vi "load data.vi"(7 "Append dataset":bool, 9 "show files":T1(array[cluster])=[{"String"="20120217.012", "Boolean"=TRUE, "begin"=15, "length"=10000, "y weight"=1.0}], 10 "existing file numbers":string[](array[string]), 11 "existing data cluster":cluster{"array type (2D Dbl)":dbl[][]}[](array[cluster])) -> (1 "show files out":T1(array[cluster])=[{"String"="20120217.012", "Boolean"=TRUE, "begin"=15, "length"=10000, "y weight"=1.0}], 2 "data names":string[](array[string]), 3 "data cluster":cluster{"all data":dbl[][]}[](array[cluster]))   [LabVIEW 2025]
uses:
  <vilib>/Utility/file.llb/Read Delimited Spreadsheet (DBL).vi
panel:
  in  "data view":bool
  in  "Done":bool
  out "# of datasets":i32
  in  "numbered file":T2={"FILE HEADER"="20120217", "FROM"="012", "TO"="012", "Excluding\nFrom"="", "Excluding\nTo"="", "Start Loading\ndata files"=FALSE, "cancel"=FALSE}
  in  "Cancel button":bool
  in  "Import Menu":T3(ring)
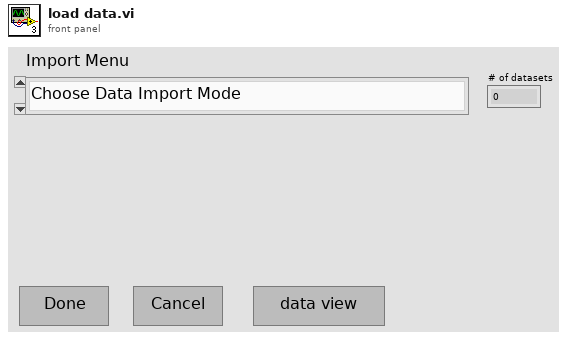
[diagram p1: front panel]
types:
  T1 = cluster{"String":string, "Boolean":bool, "begin":u32, "length":u32, "y weight":dbl}[]
  T2 = cluster{"FILE HEADER":string, "FROM":string, "TO":string, "Excluding\nFrom":string, "Excluding\nTo":string, "Start Loading\ndata files":bool, "cancel":bool}
  T3 = enum16{"Choose Data Import Mode", "Numbered NML Data Acq files saved in the drive", "Import current data being taken", "Manual selection of text file(s) ", "Manual Input of single XY plot(s)", "Manual Input of a worksheet", "Select files from a folder", "Delete Datasets"}
  T4 = enum16{"Choose Data Import Mode", "Numbered NML Data Acq files saved in the drive", "Import current data being taken", "Manual selection of text file(s) ", "Manual Input of single XY plot(s)", "Manual Input of a worksheet"}
  T5 = enum16{"Choose Data Import Mode", "Numbered NML Data Acq files saved in the drive", "Import current NML Data Acq being taken", "Manual selection of text file(s) ", "Manual Input of XY arrays", "Manual Input of a worksheet"}
  T6 = cluster{"String":string, "data view":bool, i32, i32, "new entry identier":dbl}
  T7 = cluster{"file name":string, "data view":bool, i32, i32, "new entry identier":dbl}
  T8 = cluster{"file name":string, "data view":bool, i32, i32, "new entry identier":dbl}[]
  T9 = cluster{"name":string, "data view":bool, i32, i32, "new entry identier":dbl}
  T10 = cluster{"dataset name (option)":string, "data view":bool, i32, i32, "new entry identier":dbl}
  T11 = cluster{"data set names":string, "data view":bool, i32, i32, "new entry identier":dbl}
  T12 = enum16{"Left Button", "Center Button", "Right Button", "Window Close"}
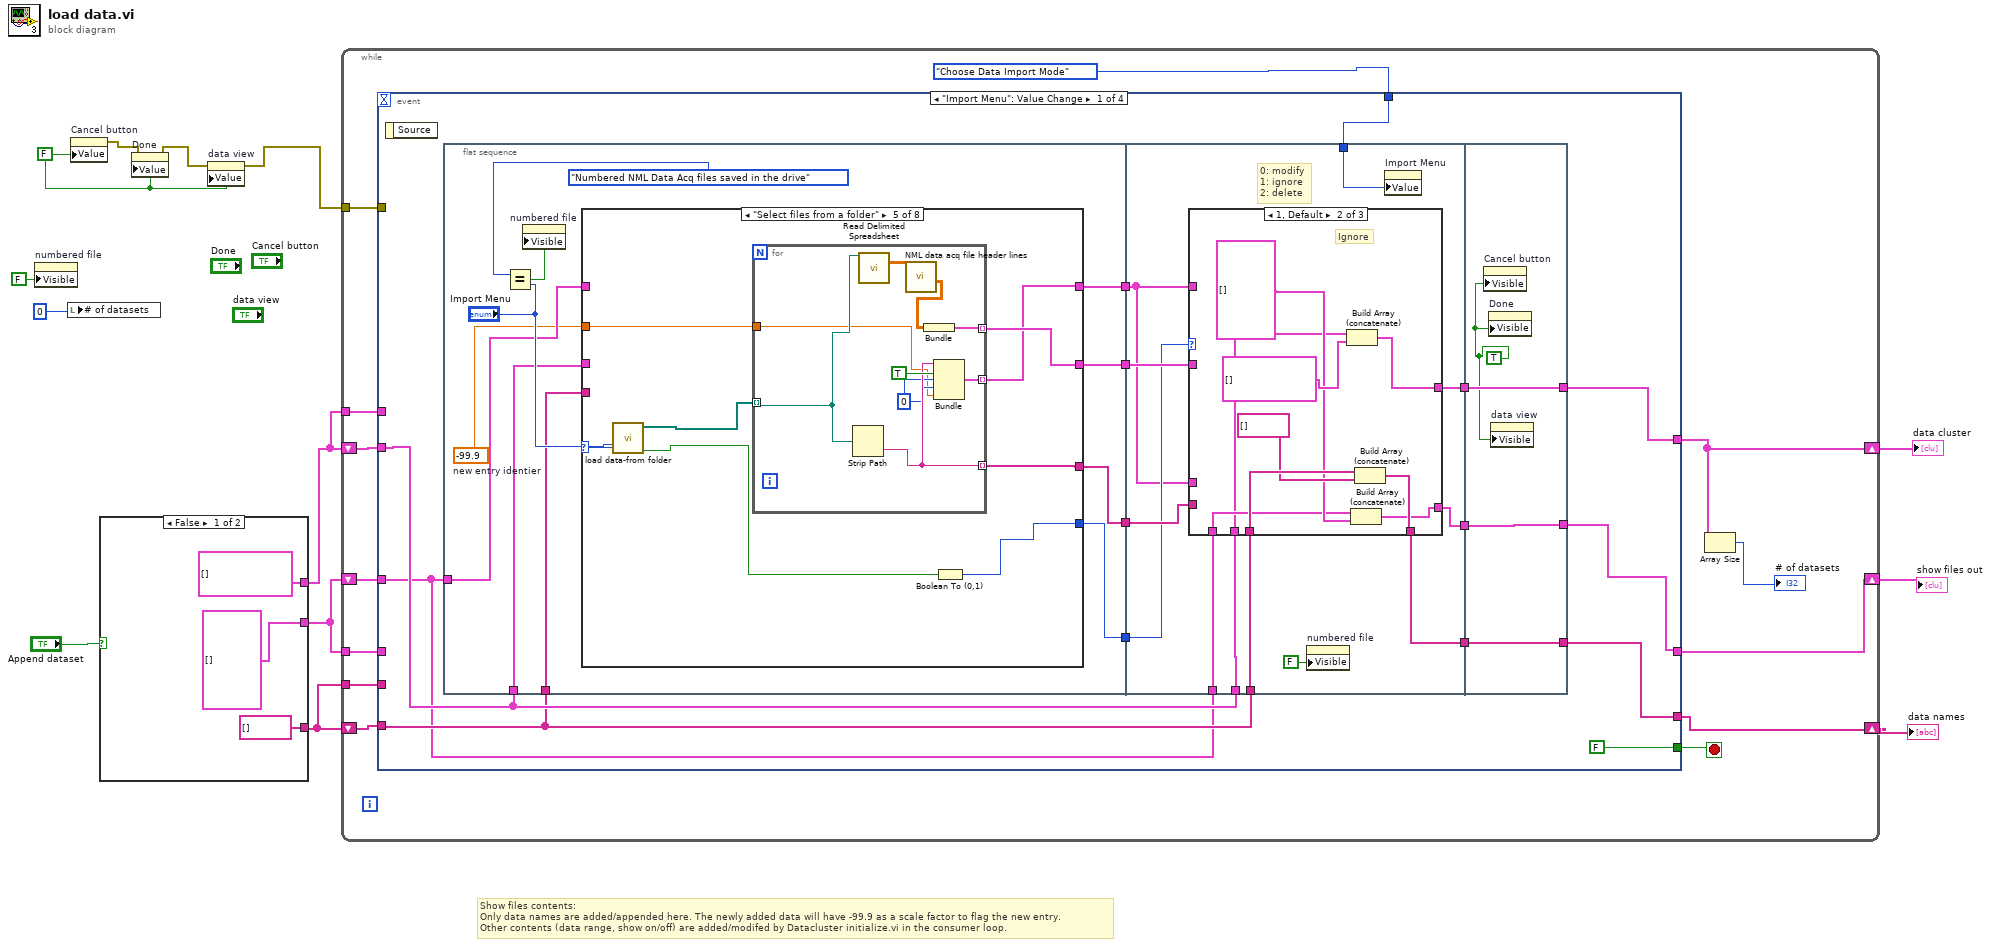
[diagram p0: block diagram]
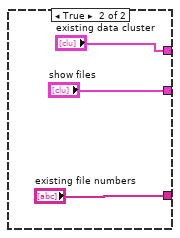
[diagram p2: hidden frame]
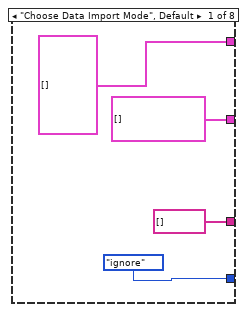
[diagram p3: hidden frame]
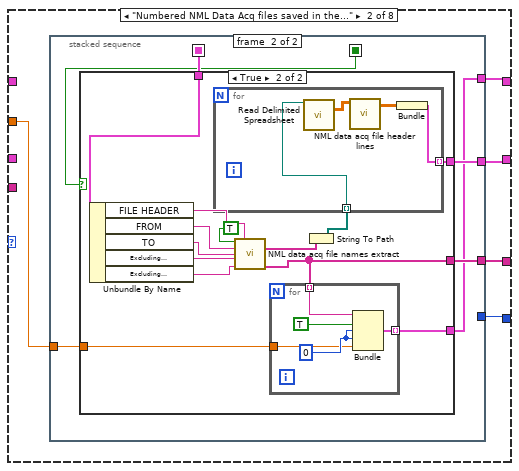
[diagram p4: hidden frame]
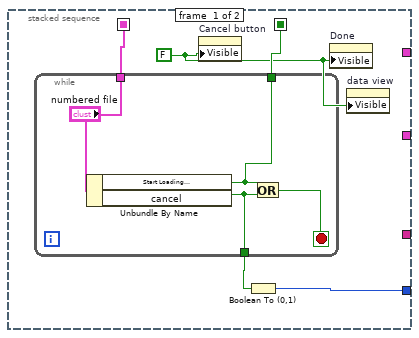
[diagram p5: hidden frame]
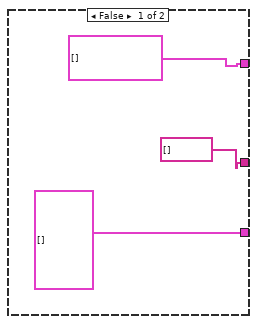
[diagram p6: hidden frame]
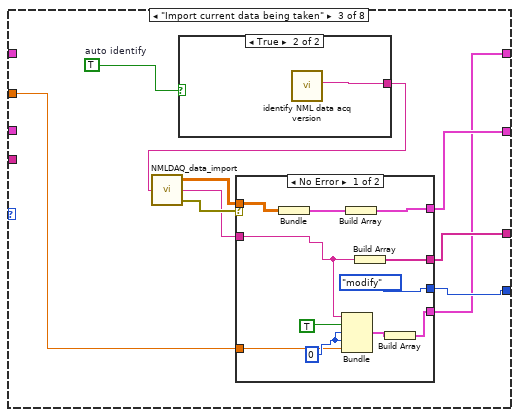
[diagram p7: hidden frame]
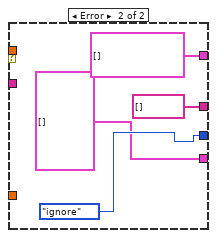
[diagram p8: hidden frame]
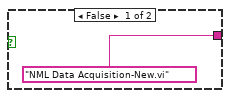
[diagram p9: hidden frame]
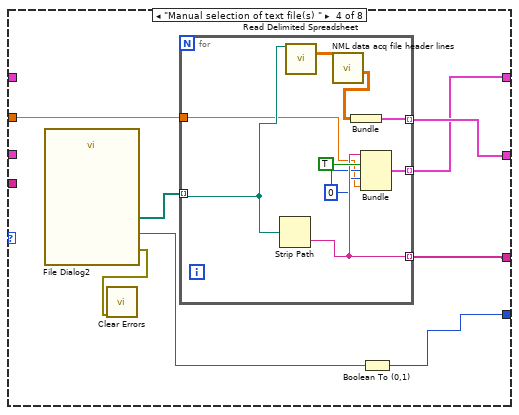
[diagram p10: hidden frame]
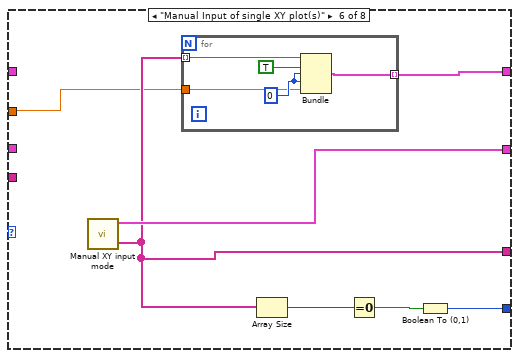
[diagram p11: hidden frame]
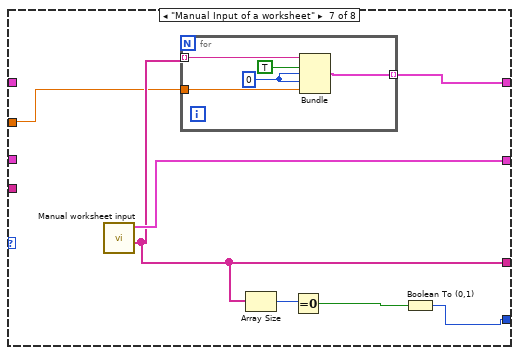
[diagram p12: hidden frame]
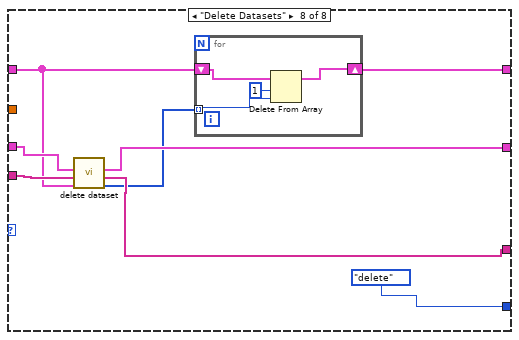
[diagram p13: hidden frame]
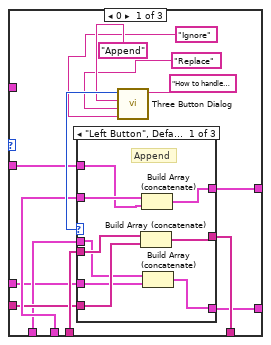
[diagram p14: hidden frame]
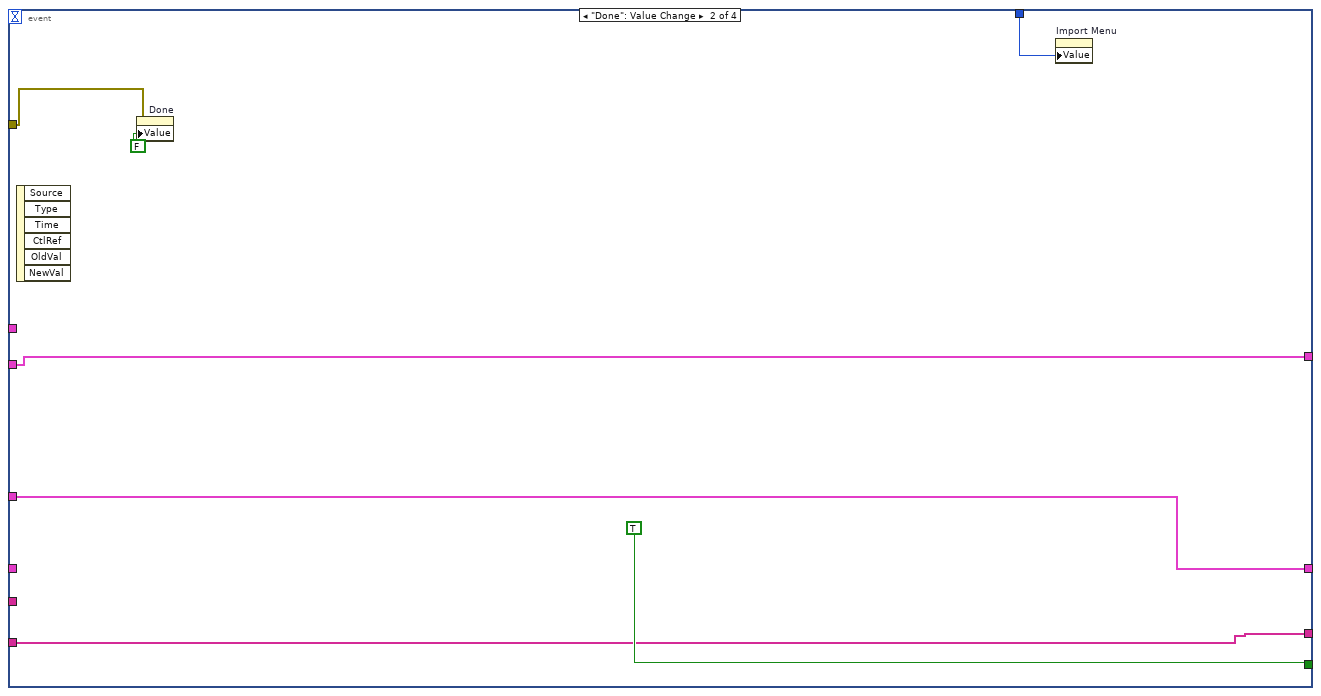
[diagram p18: hidden frame]
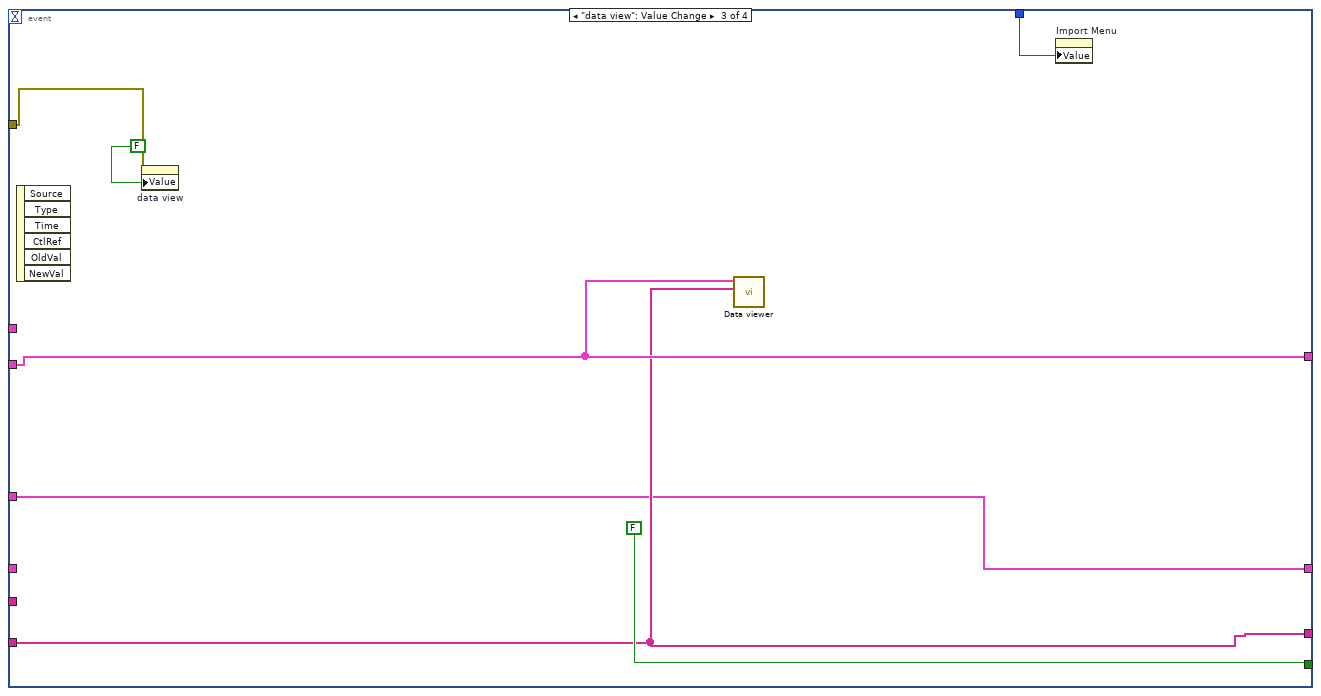
[diagram p19: hidden frame]
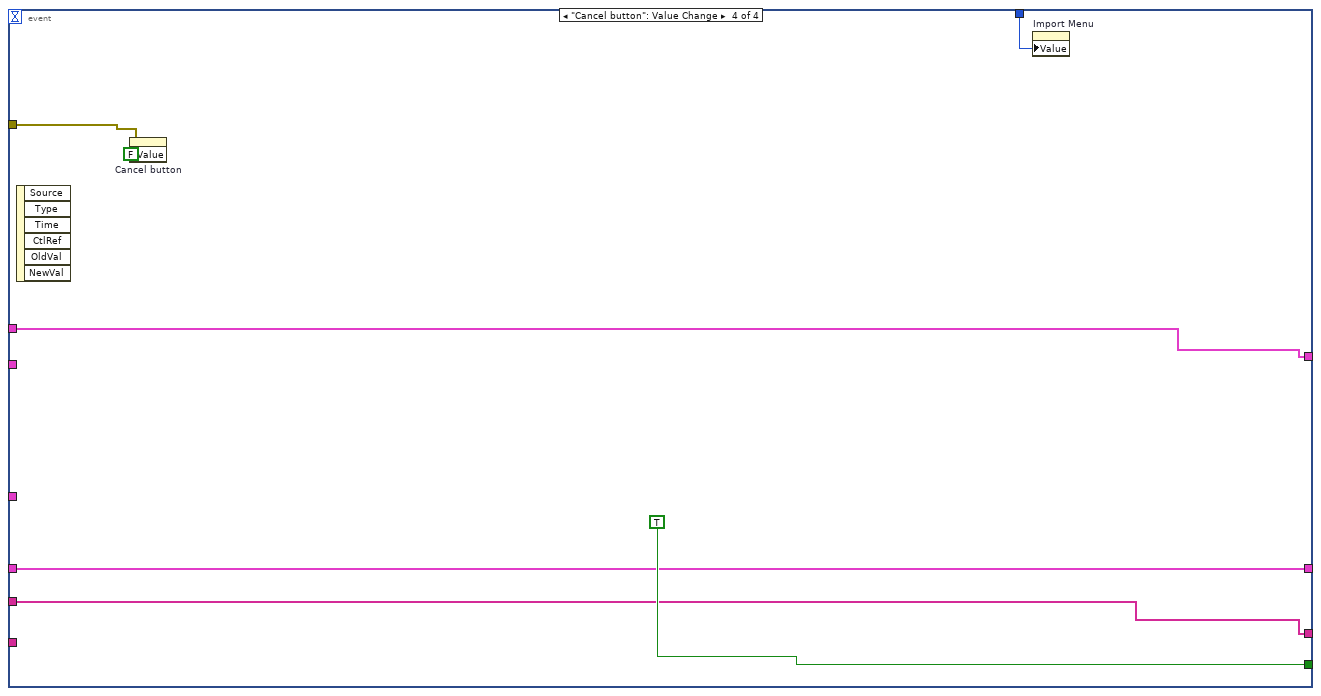
[diagram p20: hidden frame]
diagram:
  w5 = FALSE ("Value (Signaling)")
  # "Show files contents:\nOnly data names are added/appended here. The newly added data will have -99.9 as a scale factor to flag the new entry.\nOther contents (data range, show on/off) are added/modifed by Datacluster initialize.vi in the consumer loop."
  n1 = property on="numbered file" class="Clust"("Visible"=FALSE) -> ()  [unwired: 2 in, 2 out]
  n2 = local write "# of datasets"(0 ("# of data files")) -> ()
  n3 = property on="Cancel button" class="Bool (strict)"("Value"=w5) -> (error out=w8:errorcluster)  [unwired: 2 in, 1 out]
  n4 = case shown="False" "Append dataset" {
    tunnel: [cluster{"array type (2D Dbl)":dbl[][]}[] [] ("existing data cluster") "existing data cluster"] -> w4
    tunnel: [string[] [] ("existing file numbers") "existing file numbers"] -> w3
    tunnel: [T1 [] ("show files") "show files"] -> w2
    frame False {
    }
    frame True {
    }
  }
  n5 = property on="Done" class="Bool (strict)"(error in=w8, "Value"=w5) -> (error out=w7:errorcluster)  [unwired: 1 in, 1 out]
  n6 = property on="data view" class="Bool (strict)"(error in=w7, "Value"=w5) -> (error out=w6:errorcluster)  [unwired: 1 in, 1 out]
  n7 = while {
    shift-right: [w27] -> w10
    shift-left: w4 -> [w31]
    shift-right: [w28] -> w11
    shift-left: w3 -> [w29]
    tunnel: w6 -> [w26]
    tunnel: w4 -> [w24]
    tunnel: w3 -> [w23]
    shift-right: [w20] -> w1
    shift-left: w2 -> [w22]
    tunnel: w2 -> [w21]
    stop <- w32 stop-if-true
    n8 = event shown="[0] \"Import Menu\": Value Change" {
      selector: _ -> [_ _ _ _]
      dyn-events: _ -> [_ _ _ _]
      timeout: _ -> [_ _ _ _]
      tunnel: [FALSE TRUE FALSE TRUE] -> w32
      tunnel: [w46 w266 w272 w277] -> w27
      tunnel: w31 -> [w38 w266 w272 _]
      tunnel: [w45 w265 w271 w276] -> w28
      tunnel: w29 -> [w37 w265 w271 _]
      tunnel: w26 -> [_ w264 w269 w280]
      tunnel: T4."Choose Data Import Mode" ("Import Menu") -> [w44 w262 w273 w278]
      tunnel: w24 -> [_ _ _ w277]
      tunnel: w23 -> [_ _ _ w276]
      tunnel: w22 -> [w33 w261 w268 _]
      tunnel: w21 -> [_ _ _ w275]
      tunnel: [w35 w261 w268 w275] -> w20
      event "Import Menu": Value Change {
        n9 = event-data() -> ()  [unwired: 1 in, 1 out]
        n10 = flat-sequence {
          tunnel: [w56] -> w43
          tunnel: [w55] -> w42
          tunnel: [w51] -> w39
          tunnel: w38 -> [w53]
          tunnel: w37 -> [w52]
          tunnel: [w50] -> w36
          tunnel: w33 -> [w49]
          tunnel: w43 -> [w212]
          tunnel: w42 -> [w213]
          tunnel: w38 -> [w215]
          tunnel: w37 -> [w214]
          tunnel: w44 -> [w208]
          tunnel: [w211] -> w41
          tunnel: [w210] -> w40
          tunnel: w39 -> [w207]
          tunnel: w36 -> [w204]
          tunnel: [w206] -> w34
          tunnel: w33 -> [w205]
          tunnel: [w259] -> w45
          tunnel: [w260] -> w46
          tunnel: w41 -> [w260]
          tunnel: w40 -> [w259]
          tunnel: [w257] -> w35
          tunnel: w34 -> [w257]
          frame #0 {
            w48 = -99.9  # new entry identier
            n11 = Equal?(x=T5."Numbered NML Data Acq files saved in the drive", y="Import Menu") -> (x = y?=w54:bool)
            n12 = property on="numbered file" class="Clust"("Visible"=w54) -> ()  [unwired: 2 in, 2 out]
            n13 = case shown="\"Select files from a folder\"" "Import Menu" {
              tunnel: [cluster{"array type (2D Dbl)":dbl[][]}[] [] ("Data clusters") w67 w111 w142 w158 w174 w186 w196] -> w56
              tunnel: [string[] [] ("file numbers") w66 w112 w140 w157 w170 w181 w195] -> w55
              tunnel: [enum16{"modify", "ignore", "delete"}."ignore" ("Enum") w65 w110 w137 w156 w171 w183 enum16{"modify", "ignore", "delete"}."delete" ("Enum")] -> w51
              tunnel: w53 -> [_ _ _ _ _ _ _ w197]
              tunnel: w52 -> [_ _ _ _ _ _ _ w198]
              tunnel: w49 -> [_ _ _ _ _ _ _ w193]
              tunnel: [T1 [] ("show files") w64 w109 w136 w155 w169 w182 w192] -> w50
              tunnel: w48 -> [_ w63 w108 w135 w154 w168 w180 _]
              frame "Choose Data Import Mode", Default {
              }
              frame "Numbered NML Data Acq files saved in the drive" {
                n14 = stacked-sequence {
                  seq-local: [w72 _] -> [_ w81]
                  seq-local: [w71 _] -> [_ w79]
                  tunnel: [_ w82] -> w67
                  tunnel: [_ w80] -> w66
                  tunnel: [w69 _] -> w65
                  tunnel: [_ w78] -> w64
                  tunnel: w63 -> [_ w77]
                  frame #0 {
                    w68 = FALSE ("Visible")
                    n15 = while {
                      tunnel: ["numbered file"] -> w72
                      tunnel: [w74] -> w71
                      tunnel: [w73] -> w70
                      stop <- w75 stop-if-true
                      n16 = Unbundle By Name("numbered file") -> ("Start Loading\ndata files"=w74:bool, "cancel"=w73:bool)
                      n17 = Or(x=w74, y=w73) -> (x .or. y?=w75:bool)
                    }
                    n18 = property on="Cancel button" class="Bool (strict)"("Visible"=w68) -> ()  [unwired: 2 in, 2 out]
                    n19 = Boolean To (0,1)(Boolean=w70) -> (0, 1=w69:i16)
                    n20 = property on="Done" class="Bool (strict)"("Visible"=w68) -> ()  [unwired: 2 in, 2 out]
                    n21 = property on="data view" class="Bool (strict)"("Visible"=w68) -> ()  [unwired: 2 in, 2 out]
                  }
                  frame #1 {
                    n22 = case shown="True" w79 {
                      tunnel: [cluster{"array type (2D Dbl)":dbl[][]}[] [] ("Data clusters") w97] -> w82
                      tunnel: w81 -> [_ w94]
                      tunnel: [string[] [] ("file numbers") w88] -> w80
                      tunnel: [T1 [] ("show files") w87] -> w78
                      tunnel: w77 -> [_ w86]
                      frame False {
                      }
                      frame True {
                        n23 = Unbundle By Name(w94) -> ("FILE HEADER"=w93:string, "FROM"=w92:string, "TO"=w91:string, "Excluding\nFrom"=w90:string, "Excluding\nTo"=w89:string)
                        n24 = call "NML data acq file names extract.vi"("assign directory"=TRUE, "File name header"=w93, "From"=w92, "To"=w91, "Excluding From"=w90, "Excluding To"=w89) -> ("file paths"=w95:string[], "existing files"=w88:string[])  [unwired: 6 in, 2 out]
                        n25 = for {
                          tunnel: w88 -> [w102] mode=indexing
                          tunnel: [w101] -> w87 mode=indexing
                          tunnel: w86 -> [w99]
                          w100 = 0
                          n26 = Bundle("String"=w102, "data view"=TRUE, w100, w100, "new entry identier"=w99) -> (w101:T6)  [unwired: 1 in]
                        }
                        n27 = String To Path(string=w95) -> (path=w98:path[])
                        n28 = for {
                          tunnel: w98 -> [w106] mode=indexing
                          tunnel: [w107] -> w97 mode=indexing
                          n29 = call-poly <vilib>:"Read Delimited Spreadsheet.vi"("file path (dialog if empty)"=w106) -> ("all rows"=w105:dbl[][])  [unwired: 9 in, 5 out]
                          n30 = call "NML data acq file header lines.vi"("all rows"=w105) -> ("real data?"=w104:dbl[][])  [unwired: 8 in, 2 out]
                          n31 = Bundle("real data?"=w104) -> (w107:cluster{"real data?":dbl[][]})  [unwired: 1 in]
                        }
                      }
                    }
                  }
                }
              }
              frame "Import current data being taken" {
                w116 = TRUE  # auto identify
                n32 = case shown="True" w116 {
                  tunnel: ["NML Data Acquisition-New.vi" ("NML Data Acquisition VI") w134] -> w117
                  frame False {
                  }
                  frame True {
                    n33 = call "identify NML data acq version.vi"() -> ("NML data in the memory"=w134:string)  [unwired: 11 in]
                  }
                }
                n34 = call "NMLDAQ_data_import.vi"("NML Data Acquisition VI"=w117) -> ("data"=w114:dbl[][], "file name"=w113:string, "error out"=w115:errorcluster)
                n35 = case shown="No Error" w115 {
                  tunnel: w114 -> [w121 _]
                  tunnel: w113 -> [w124 _]
                  tunnel: [w127 string[] []] -> w112
                  tunnel: [w126 cluster{"data":dbl[][]}[] []] -> w111
                  tunnel: [enum16{"modify", "ignore", "delete"}."modify" ("Enum") enum16{"modify", "ignore", "delete"}."ignore" ("Enum")] -> w110
                  tunnel: [w120 T1 [] ("show files")] -> w109
                  tunnel: w108 -> [w118 _]
                  frame No Error {
                    w119 = 0
                    n36 = Bundle("data"=w121) -> (w128:cluster{"data":dbl[][]})  [unwired: 1 in]
                    n37 = Bundle("file name"=w124, "data view"=TRUE, w119, w119, "new entry identier"=w118) -> (w122:T7)  [unwired: 1 in]
                    n38 = Build Array(w128) -> (w126:cluster{"data":dbl[][]}[])
                    n39 = Build Array(w124) -> (w127:string[])
                    n40 = Build Array(w122) -> (w120:T8)
                  }
                  frame Error {
                  }
                }
              }
              frame "Manual selection of text file(s) " {
                n41 = call "File Dialog2"() -> ("selected paths"=w141:path[], "cancelled"=w138:bool, "error out"=w139:errorcluster)  [unwired: 12 in, 1 out]
                n42 = call <vilib>:"Clear Errors.vi"("error in (no error)"=w139) -> ()  [unwired: 5 in, 2 out]
                n43 = for {
                  tunnel: w141 -> [w150] mode=indexing
                  tunnel: [w151] -> w142 mode=indexing
                  tunnel: [w146] -> w140 mode=indexing
                  tunnel: [w145] -> w136 mode=indexing
                  tunnel: w135 -> [w143]
                  w144 = 0
                  n44 = Strip Path(path=w150) -> (name=w146:string)  [unwired: 1 out]
                  n45 = call-poly <vilib>:"Read Delimited Spreadsheet.vi"("file path (dialog if empty)"=w150) -> ("all rows"=w149:dbl[][])  [unwired: 9 in, 5 out]
                  n46 = call "NML data acq file header lines.vi"("all rows"=w149) -> ("real data?"=w148:dbl[][])  [unwired: 8 in, 2 out]
                  n47 = Bundle("real data?"=w148) -> (w151:cluster{"real data?":dbl[][]})  [unwired: 1 in]
                  n48 = Bundle("name"=w146, "data view"=TRUE, w144, w144, "new entry identier"=w143) -> (w145:T9)  [unwired: 1 in]
                }
                n49 = Boolean To (0,1)(Boolean=w138) -> (0, 1=w137:i16)
              }
              frame "Select files from a folder" {
                n50 = call "load data-from folder.vi"() -> ("cancelled"=w152:bool, "selected files"=w153:path[])  [unwired: 10 in]
                n51 = for {
                  tunnel: w153 -> [w166] mode=indexing
                  tunnel: [w167] -> w158 mode=indexing
                  tunnel: [w162] -> w157 mode=indexing
                  tunnel: [w161] -> w155 mode=indexing
                  tunnel: w154 -> [w159]
                  w160 = 0
                  n52 = Strip Path(path=w166) -> (name=w162:string)  [unwired: 1 out]
                  n53 = call-poly <vilib>:"Read Delimited Spreadsheet.vi"("file path (dialog if empty)"=w166) -> ("all rows"=w165:dbl[][])  [unwired: 9 in, 5 out]
                  n54 = call "NML data acq file header lines.vi"("all rows"=w165) -> ("real data?"=w164:dbl[][])  [unwired: 8 in, 2 out]
                  n55 = Bundle("real data?"=w164) -> (w167:cluster{"real data?":dbl[][]})  [unwired: 1 in]
                  n56 = Bundle("name"=w162, "data view"=TRUE, w160, w160, "new entry identier"=w159) -> (w161:T9)  [unwired: 1 in]
                }
                n57 = Boolean To (0,1)(Boolean=w152) -> (0, 1=w156:i16)
              }
              frame "Manual Input of single XY plot(s)" {
                n58 = call "Manual XY input mode.vi"() -> ("Data clusters"=w174:cluster{"array type (2D Dbl)":dbl[][]}[], "data names"=w170:string[])  [unwired: 7 in, 3 out]
                n59 = for {
                  tunnel: w170 -> [w178] mode=indexing
                  tunnel: [w177] -> w169 mode=indexing
                  tunnel: w168 -> [w175]
                  w176 = 0
                  n60 = Bundle("dataset name (option)"=w178, "data view"=TRUE, w176, w176, "new entry identier"=w175) -> (w177:T10)  [unwired: 1 in]
                }
                n61 = Array Size(array=w170) -> (size(s)=w173:i32)
                n62 = Equal To 0?(x=w173) -> (x = 0?=w172:bool)
                n63 = Boolean To (0,1)(Boolean=w172) -> (0, 1=w171:i16)
              }
              frame "Manual Input of a worksheet" {
                n64 = call "Manual worksheet input.vi"() -> ("data names"=w181:string[], "Data clusters"=w186:cluster{"array type (2D Dbl)":dbl[][]}[])  [unwired: 8 in, 2 out]
                n65 = for {
                  tunnel: w181 -> [w190] mode=indexing
                  tunnel: [w189] -> w182 mode=indexing
                  tunnel: w180 -> [w187]
                  w188 = 0
                  n66 = Bundle("data set names"=w190, "data view"=TRUE, w188, w188, "new entry identier"=w187) -> (w189:T11)  [unwired: 1 in]
                }
                n67 = Array Size(array=w181) -> (size(s)=w185:i32)
                n68 = Equal To 0?(x=w185) -> (x = 0?=w184:bool)
                n69 = Boolean To (0,1)(Boolean=w184) -> (0, 1=w183:i16)
              }
              frame "Delete Datasets" {
                n70 = call "delete dataset.vi"("show files"=w193, "existing file numbers"=w198, "existing data cluster"=w197) -> ("deleted"=w194:i32[], "survived dataset names"=w195:string[], "survived dataset"=w196:cluster{"array type (2D Dbl)":dbl[][]}[])  [unwired: 4 in]
                n71 = for {
                  shift-right: [w200] -> w192
                  shift-left: w193 -> [w203]
                  tunnel: w194 -> [w202] mode=indexing
                  n72 = Delete From Array(array=w203, length=1, index=w202) -> (array with subset deleted=w200:T1)  [unwired: 1 out]
                }
              }
            }
          }
          frame #1 {
            # "0: modify\n1: ignore\n2: delete"
            n73 = case shown="1, Default" w207 {
              tunnel: w215 -> [w224 w245 _]
              tunnel: w214 -> [w223 w251 _]
              tunnel: w213 -> [w222 _ w255]
              tunnel: w212 -> [w221 _ w256]
              tunnel: [w220 w252 w256] -> w211
              tunnel: [w219 w249 w255] -> w210
              tunnel: w204 -> [_ _ w254]
              tunnel: [w218 w246 w254] -> w206
              tunnel: w205 -> [w217 w247 _]
              tunnel: w204 -> [w216 _ _]
              frame 0 {
                n74 = call <vilib>:"Three Button Dialog.vi"("Right Button Text (\"Cancel\")"="Ignore" ("Right Button Text (\"Cancel\")"), "Center Button Text (\"No\")"="Replace" ("Center Button Text (\"No\")"), "Left Button Text (\"Yes\")"="Append" ("Left Button Text (\"Yes\")"), "message"="How to handle the imported data?") -> ("Which Button?"=w229:T12)  [unwired: 7 in]
                n75 = case shown="\"Left Button\", Default" w229 {
                  tunnel: [w238 w241 w244] -> w220
                  tunnel: [w237 w240 w243] -> w219
                  tunnel: w224 -> [w236 _ w244]
                  tunnel: w223 -> [w235 _ w243]
                  tunnel: w222 -> [w234 w240 _]
                  tunnel: w221 -> [w233 w241 _]
                  tunnel: [w230 w239 w242] -> w218
                  tunnel: w217 -> [w231 _ w242]
                  tunnel: w216 -> [w232 w239 _]
                  frame "Left Button", Default {
                    # "Append"
                    n76 = Build Array (concatenate)(w235, w234) -> (w237:string[])
                    n77 = Build Array (concatenate)(w236, w233) -> (w238:cluster{"array type (2D Dbl)":dbl[][]}[])
                    n78 = Build Array (concatenate)(w231, w232) -> (w230:T1)
                  }
                  frame "Center Button" {
                    # "Replace"
                  }
                  frame "Right Button" {
                    # "Ignore"
                  }
                }
              }
              frame 1, Default {
                # "Ignore"
                n79 = Build Array (concatenate)(w245, cluster{"array type (2D Dbl)":dbl[][]}[] []) -> (w252:cluster{"array type (2D Dbl)":dbl[][]}[])
                n80 = Build Array (concatenate)(w247, T1 [] ("show files")) -> (w246:T1)
                n81 = Build Array (concatenate)(w251, string[] []) -> (w249:string[])
              }
              frame 2 {
                # "data and show files\nare managed in the previous\nframe"
              }
            }
            n82 = property on="numbered file" class="Clust"("Visible"=FALSE) -> ()  [unwired: 2 in, 2 out]
            n83 = property on="Import Menu" class="Enum (strict)"("Value"=w208) -> ()  [unwired: 2 in, 2 out]
          }
          frame #2 {
            w258 = TRUE ("Visible")
            n84 = property on="Cancel button" class="Bool (strict)"("Visible"=w258) -> ()  [unwired: 2 in, 2 out]
            n85 = property on="Done" class="Bool (strict)"("Visible"=w258) -> ()  [unwired: 2 in, 2 out]
            n86 = property on="data view" class="Bool (strict)"("Visible"=w258) -> ()  [unwired: 2 in, 2 out]
          }
        }
      }
      event "Done": Value Change {
        n87 = event-data() -> ()  [unwired: 1 in, 6 out]
        n88 = property on="Done" class="Bool (strict)"(error in=w264, "Value"=FALSE ("Value (Signaling)")) -> ()  [unwired: 1 in, 2 out]
        n89 = property on="Import Menu" class="Enum (strict)"("Value"=w262) -> ()  [unwired: 2 in, 2 out]
      }
      event "data view": Value Change {
        n90 = event-data() -> ()  [unwired: 1 in, 6 out]
        n91 = property on="data view" class="Bool (strict)"(error in=w269, "Value"=FALSE ("Value (Signaling)")) -> ()  [unwired: 1 in, 2 out]
        n92 = call "Data viewer.vi"("data names"=w271, "data cluster"=w272) -> ()  [unwired: 10 in]
        n93 = property on="Import Menu" class="Enum (strict)"("Value"=w273) -> ()  [unwired: 2 in, 2 out]
      }
      event "Cancel button": Value Change {
        n94 = event-data() -> ()  [unwired: 1 in, 6 out]
        n95 = property on="Cancel button" class="Bool (strict)"(error in=w280, "Value"=FALSE ("Value (Signaling)")) -> ()  [unwired: 1 in, 2 out]
        n96 = property on="Import Menu" class="Enum (strict)"("Value"=w278) -> ()  [unwired: 2 in, 2 out]
      }
    }
    n97 = Array Size(array=w27) -> (size(s)=→"# of datasets":i32)
  }
  "data cluster" <- w10
  "data names" <- w11
  "show files out" <- w1
